vi "WT-Voltage-Controller-Current.vi"() -> ()   [LabVIEW 2016]
uses:
  <vilib>/Platform/TimedLoop/XDataNode/timing_clust.ctl
  <vilib>/Platform/TimedLoop/XDataNode/nitl_modes.ctl
  <vilib>/Platform/TimedLoop/XDataNode/wakeup.ctl
  <vilib>/DAQmx/read.llb/DAQmx Read (Analog 1D DBL NChan 1Samp).vi
  <vilib>/Analysis/baseanly.llb/Mean (DBL).vi
  <vilib>/DAQmx/miscellaneous.llb/DAQmx Fill In Error Info.vi
  <vilib>/platform/TimedLoop/XDataNode/XDataNode.xnode
  <vilib>/Platform/TimedLoop/XDataNode/XDNodeRunTimeDep.lvlib
  <vilib>/Analysis/NI_AALBase.lvlib
panel:
  out "Fan 2 (A)":dbl format="%0.2f"
  out "Fan 1 (A)":dbl format="%0.2f"
  out "Boolean":bool
  in  "POWER":bool
  in  "Sync":bool
  out "error out":errorcluster
  in  "Fan 2 Voltage":dbl(knob) scale=0.0..10.0
  in  "Fan 1 Voltage":dbl(knob) scale=0.0..10.0
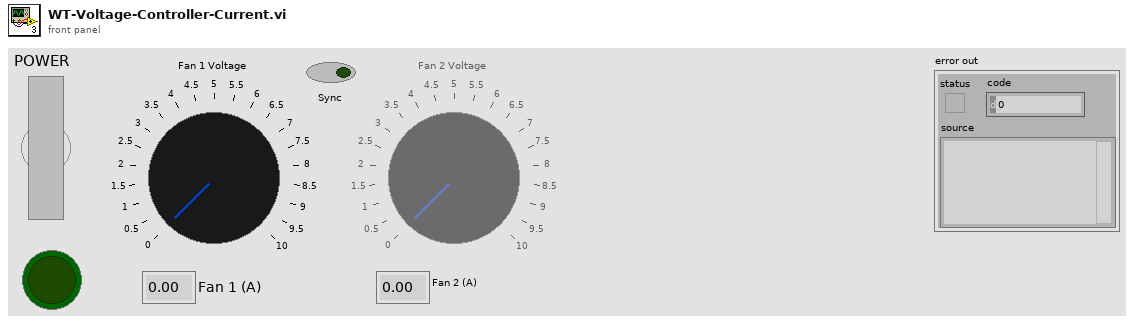
[diagram p1: front panel]
types:
  T1 = typedef "XDNodeRunTimeDep.lvlib/timing_clust.ctl" = cluster{"Expected End [f-1]":u64, "Actual End [f-1]":u64, "Finished Late? [f-1]":bool, "Expected End [i-1]":u64, "Actual End [i-1]":u64, "Finished Late? [i-1]":bool, "Expected Start [i]":u64, "Actual Start [i]":u64, "Expected Start [f]":u64, "Actual Start [f]":u64, "Source Name":string, "Structure Name":string, "Period":i64, "Deadline":i64, "Offset":i64, "Start":i64, "Priority":i32, "Timeout":i32, "Mode":T2, "Wakeup Reason":T3, "Error":errorcluster, "Source Type":string, "Secondary Source Type":string, "Global End Time":u64, "Global Start Time":u64, "Frame Duration":u64, "Iteration Duration":u64, "Assigned CPU":i32, "I/O Scan Engine Mode":u32}
  T2 = typedef "XDNodeRunTimeDep.lvlib/nitl_modes.ctl" = enum32{"No Change", "Process missed periods, maintain original phase", "Discard missed periods, maintain original phase", "Process missed periods, ignore original phase", "Discard missed periods, ignore original phase"}
  T3 = typedef "XDNodeRunTimeDep.lvlib/wakeup.ctl" = enum32{"Normal", "Aborted", "Asynchronous wakeup", "Timing source error", "Timed loop error", "Timeout"}
  T4 = enum8{"Enabled", "Disabled", "Disabled and Grayed Out"}
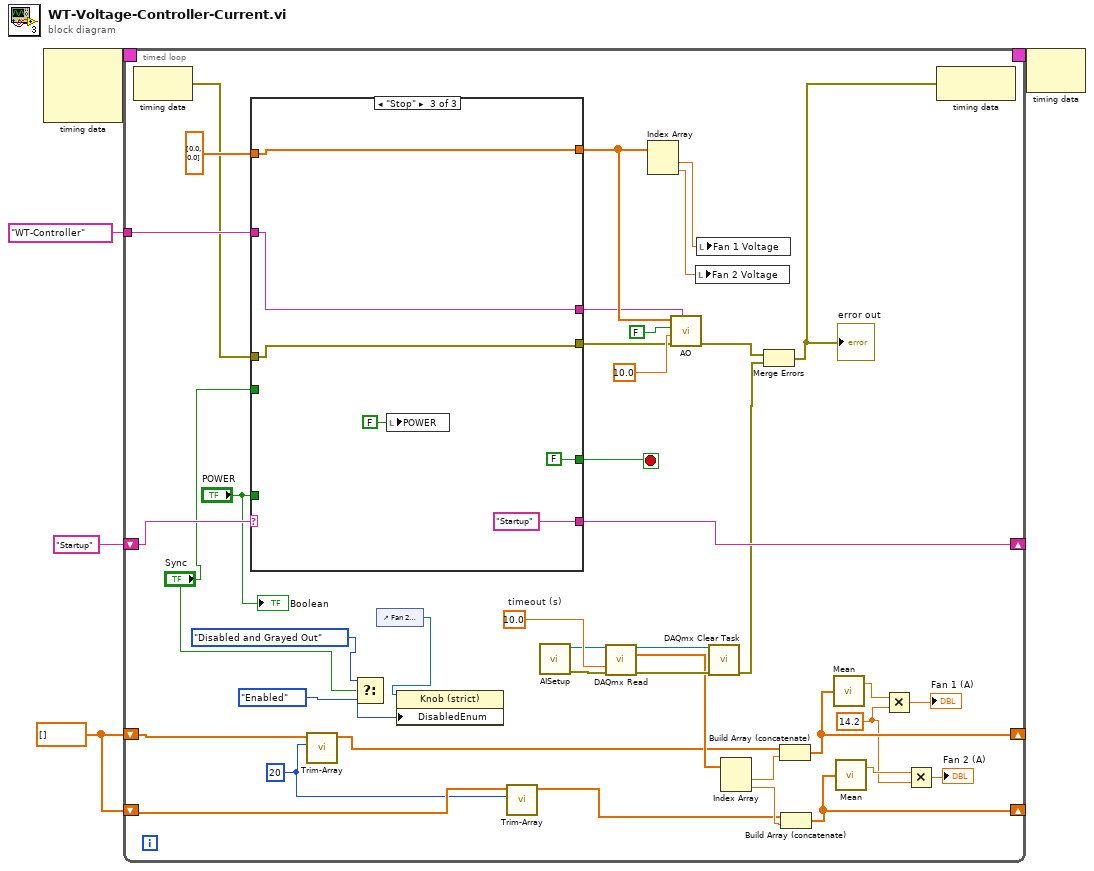
[diagram p0: block diagram]
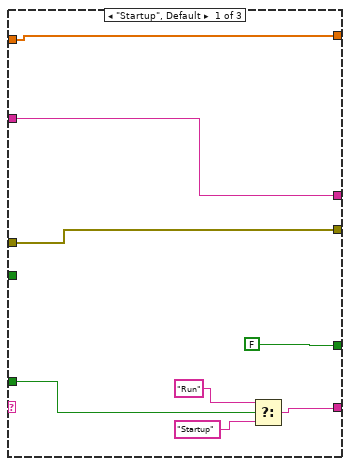
[diagram p2: hidden frame]
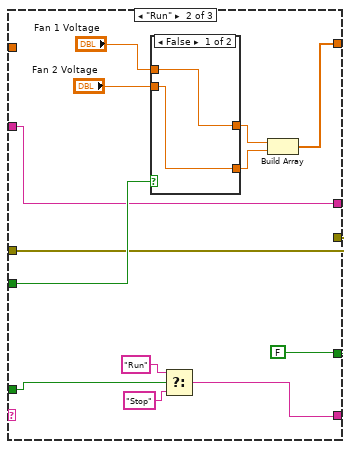
[diagram p3: hidden frame]
diagram:
  w1 = dbl[] []
  n1 = node-c288() -> (w3:T1)  [unwired: 3 in]
  n2 = timed-loop {
    shift-right: [w46] -> _
    shift-left: "Startup" -> [w47]
    tunnel: tag "WT-Controller" ("device name") -> [w44]
    timing: w3 -> [_]
    timing-out: [_] -> w2
    shift-right: [w16] -> _
    shift-left: w1 -> [w14]
    shift-right: [w15] -> _
    shift-left: w1 -> [w13]
    stop <- w45 stop-if-true
    w7 = 14.2 ("y")
    w11 = 20 ("length")
    w28 = 10.0  # timeout (s)
    n3 = node-c288() -> (w33:errorcluster)  [unwired: 1 in]
    n4 = case shown="\"Stop\"" w47 {
      tunnel: [w54 w73 "Startup" ("f")] -> w46
      tunnel: [w59 w66 w80] -> w37
      tunnel: [FALSE ("Stop") FALSE ("Stop") FALSE ("Stop")] -> w45
      tunnel: w44 -> [w58 w65 w81]
      tunnel: [w60 w64 w79] -> w35
      tunnel: w33 -> [w60 w64 w79]
      tunnel: "Sync" -> [_ w68 _]
      tunnel: dbl[] [0.0, 0.0] ("appended array") -> [w59 _ w80]
      tunnel: [w58 w65 w81] -> w34
      tunnel: "POWER" -> [w56 w63 _]
      frame "Startup", Default {
        n5 = Select(t="Run" ("f"), s=w56, f="Startup") -> (s? t:f=w54:string)
      }
      frame "Run" {
        n6 = case shown="False" w68 {
          tunnel: [w74 w76] -> w71
          tunnel: [w75 w76] -> w70
          tunnel: "Fan 1 Voltage" -> [w75 w76]
          tunnel: "Fan 2 Voltage" -> [w74 _]
          frame False {
          }
          frame True {
          }
        }
        n7 = Select(t="Run" ("f"), s=w63, f="Stop") -> (s? t:f=w73:string)
        n8 = Build Array(w70, w71) -> (w66:dbl[])
      }
      frame "Stop" {
        n9 = local write "POWER"(FALSE ("POWER")) -> ()
      }
    }
    n10 = call "Trim-Array.vi"("length"=w11, "Array in"=w14) -> ("Array out"=w18:dbl[])  [unwired: 9 in]
    n11 = Select(t=T4."Disabled and Grayed Out" ("Disabled"), s="Sync", f=T4."Enabled") -> (s? t:f=w42:T4)
    n12 = control-ref of="Fan 2 Voltage"() -> (w40:refnum<vi>)
    n13 = property class="Knob (strict)"(reference=w40, "DisabledEnum"=w42) -> ()  [unwired: 1 in, 2 out]
    n14 = call "Trim-Array.vi"("length"=w11, "Array in"=w13) -> ("Array out"=w12:dbl[])  [unwired: 9 in]
    n15 = call "AISetup.vi"() -> ("error out"=w24:errorcluster, "task out"=w25:refnum<k21>)  [unwired: 10 in]
    n16 = call-poly <vilib>:"DAQmx Read.vi"("task/channels in"=w25, "timeout"=w28, "error in"=w24) -> ("task out"=w26:refnum<k21>, "data"=w20:dbl[], "error out"=w27:errorcluster)  [unwired: 10 in]
    n17 = Index Array(array=w37) -> (element #1=w32:dbl, element #2=w31:dbl)  [unwired: 2 in]
    n18 = call "AO.vi"("device name"=w34, "error in"=w35, "timeout (s)"=10.0, "stop (T)"=FALSE, "data"=w37) -> ("error out"=w22:errorcluster)  [unwired: 2 in, 1 out]
    n19 = local write "Fan 2 Voltage"(w31) -> ()
    n20 = local write "Fan 1 Voltage"(w32) -> ()
    n21 = call <vilib>:"DAQmx Clear Task.vi"("task in"=w26, "error in"=w27) -> ("error out"=w23:errorcluster)  [unwired: 13 in]
    n22 = Index Array(array=w20) -> (element #1=w19:dbl, element #2=w17:dbl)  [unwired: 2 in]
    n23 = Merge Errors(w22, w23) -> (w21:errorcluster)
    "error out" <- w21
    n24 = Build Array (concatenate)(w18, w19) -> (w16:dbl[])
    n25 = Build Array (concatenate)(w12, w17) -> (w15:dbl[])
    n26 = call-poly <vilib>:"Mean.vi"("X"=w16) -> ("mean"=w10:dbl)  [unwired: 1 out]
    n27 = call-poly <vilib>:"Mean.vi"("X"=w15) -> ("mean"=w8:dbl)  [unwired: 1 out]
    n28 = Multiply(x=w10, y=w7) -> (x*y=→"Fan 1 (A)":dbl)
    n29 = Multiply(x=w8, y=w7) -> (x*y=→"Fan 2 (A)":dbl)
    n30 = node-c288(w21) -> ()  [unwired: 1 out]
    "Boolean" <- "POWER"
  }
  n31 = node-c288(w2) -> ()  [unwired: 1 out]
